vi "Read Default Settings.vi"(8 "error in (no error)":errorcluster, 11 "Application in":refnum<class "Application.lvclass">) -> (0 "error out":errorcluster, 2 "Default Settings":T1={"Refresh Timeout (ms)"=100, "Version String"="", "Hardware Configuration File"=""}, 3 "Application out":refnum<class "Application.lvclass">)   [LabVIEW 2015, in "Application.lvlib" / "Application.lvclass"]
uses:
  Application.lvclass
  Resources/Type Defs/Default Settings.ctl
  Application.lvclass/Application.ctl
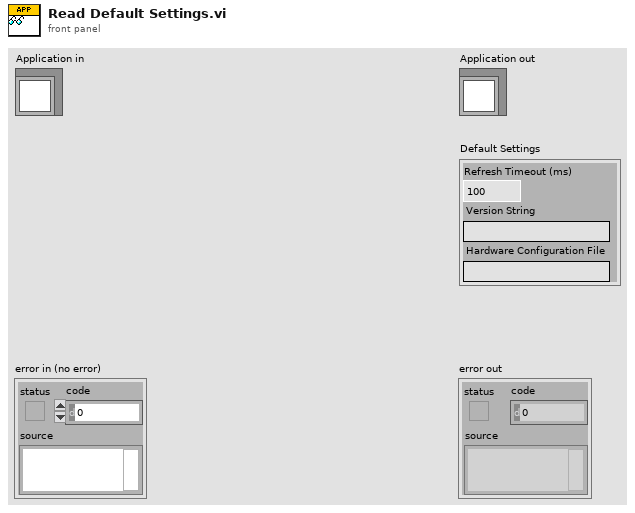
[diagram p1: front panel]
types:
  T1 = typedef "Default Settings.ctl" = cluster{"Refresh Timeout (ms)":i32, "Version String":string, "Hardware Configuration File":string}
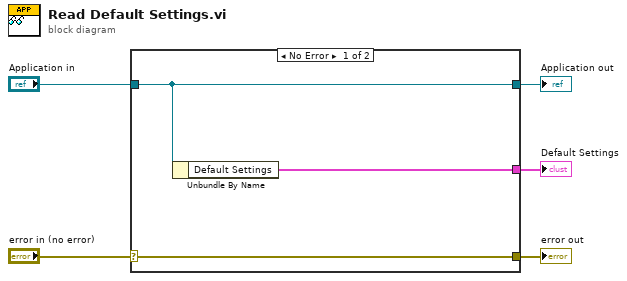
[diagram p0: block diagram]
diagram:
  n1 = case shown="No Error" "error in (no error)" {
    selector: "error in (no error)" -> [w8 w9]
    tunnel: [w8 w9] -> w4
    tunnel: [w7 w10] -> w2
    tunnel: "Application in" -> [w7 w10]
    tunnel: [w6 _] -> w1
    frame No Error {
      n2 = Unbundle By Name(w7) -> ("Default Settings"=w6:T1)
    }
    frame Error {
    }
  }
  "error out" <- w4
  "Application out" <- w2
  "Default Settings" <- w1
